vi "简单工厂模式客户端(包含初始化).vi"() -> ()   [LabVIEW 2013]
panel:
  out "运算结果":dbl
  in  "输入B":dbl
  in  "输入A":dbl
  in  "运算":T1
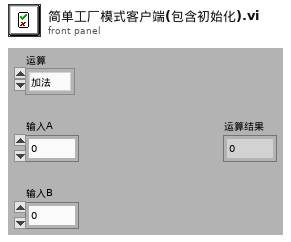
[diagram p1: front panel]
types:
  T1 = typedef "运算工厂.lvclass/运算方法.ctl" = enum16{"加法", "减法", "乘法", "平方和"}
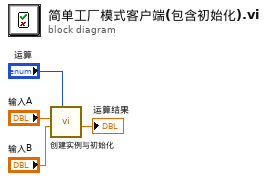
[diagram p0: block diagram]
diagram:
  n1 = call "创建实例与初始化.vi"("运算"="运算", "B"="输入B", "A"="输入A") -> ("结果"=→"运算结果":dbl)  [unwired: 5 in, 3 out]
